vi "Dialogue_visa_GFS4470_Emballage_BDD.vi"(6 "entrée d'erreur (pas d'erreur)":errorcluster, 9 "nom de ressource VISA":refnum<visa-resource-name>="ASRL3::INSTR") -> (0 "error out":errorcluster, 3 "buffer lu":string)   [LabVIEW 2020]
uses:
  Modules/FS/60_FS_Controles/60_FS_SetGet.ctl
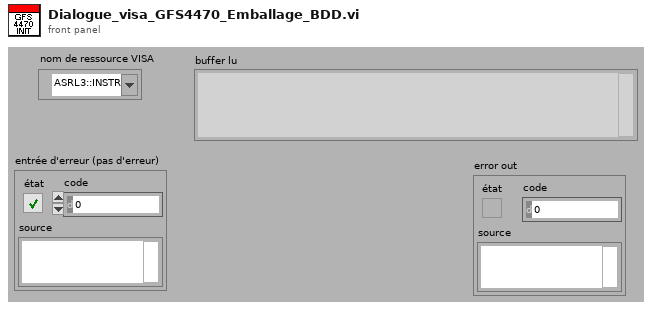
[diagram p1: front panel]
types:
  T1 = typedef "60_FS_SetGet.ctl" = enum16{"set", "get"}
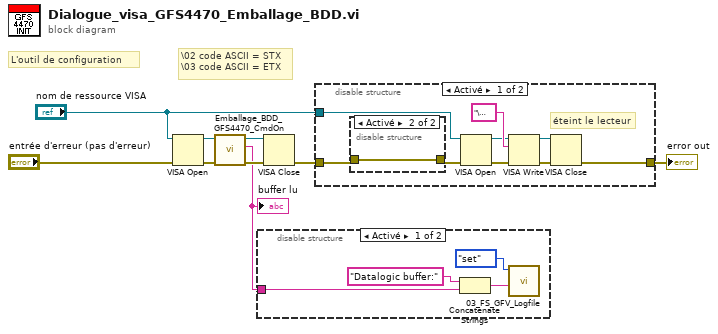
[diagram p0: block diagram]
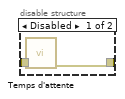
[diagram p3: hidden frame]
diagram:
  # "L'outil de configuration"
  # "\\02 code ASCII = STX\n\\03 code ASCII = ETX"
  n1 = VISA Open(error in (no error)="entrée d'erreur (pas d'erreur)", VISA resource name="nom de ressource VISA") -> (VISA resource name=w5:refnum<visa-resource-name>, error out=w4:errorcluster)  [unwired: 3 in]
  n2 = call "Emballage_BDD_GFS4470_CmdOn.vi"("error in (no error)"=w4, "VISA Datalogic 5"=w5) -> ("sortie d'erreur"=w3:errorcluster, "buffer de lecture"=w1:string, "Nom de ressource VISA en sortie"=w2:refnum<visa-resource-name>)  [unwired: 6 in, 1 out]
  "buffer lu" <- w1
  n3 = disable-structure shown="Activé" {
    disable-tunnel: w1 -> [w10 _]
    frame Enabled {
      n4 = Concatenate Strings("Datalogic buffer:" ("Chaîne"), w10) -> (w12:string)
      n5 = call "03_FS_GFV_Logfile.vi"("Chaîne"=w12, "States"=60_FS_SetGet."set") -> ()  [unwired: 8 in, 2 out]
    }
    frame Disabled {
    }
  }
  n6 = VISA Close(VISA resource name=w2, error in (no error)=w3) -> (error out=w8:errorcluster)
  n7 = disable-structure shown="Activé" {
    disable-tunnel: "nom de ressource VISA" -> [w17 _]
    disable-tunnel: w8 -> [w16 w26]
    disable-tunnel: [w14 w26] -> w7
    frame Enabled {
      # "éteint le lecteur"
      n8 = disable-structure shown="Activé" {
        disable-tunnel: w16 -> [w24 w25]
        disable-tunnel: [w23 w25] -> w15
        frame Disabled {
          n9 = call "Temps d'attente"("error in (no error)"=w24) -> ("error out"=w23:errorcluster)  [unwired: 10 in]
        }
        frame Enabled {
        }
      }
      n10 = VISA Open(error in (no error)=w15, VISA resource name=w17) -> (VISA resource name=w19:refnum<visa-resource-name>, error out=w21:errorcluster)  [unwired: 3 in]
      n11 = VISA Write(VISA resource name=w19, write buffer="\u0003", error in (no error)=w21) -> (VISA resource name out=w18:refnum<visa-resource-name>, error out=w20:errorcluster)  [unwired: 1 out]
      n12 = VISA Close(VISA resource name=w18, error in (no error)=w20) -> (error out=w14:errorcluster)
    }
    frame Disabled {
    }
  }
  "error out" <- w7
